vi "Set Path.vi"(7 "Use base-path?":bool, 8 "error in (no error)":errorcluster, 9 "Encode?":bool, 10 "path":string, 11 "URI in":refnum<class "URI.lvclass">) -> (0 "error out":errorcluster, 3 "URI out":refnum<class "URI.lvclass">)   [LabVIEW 2013, in "openURI.lvlib" / "URI.lvclass"]
uses:
  URI.lvclass
  URI.lvclass/URI.ctl
  utilities/isHEXDigit.vi
  components/path/Get base-path.vi
  components/path/Create Path (string).vi
  <vilib>/Utility/error.llb/Error Cluster From Error Code.vi
  checkCached.vi
  components/path/URI-Component.Path.lvclass
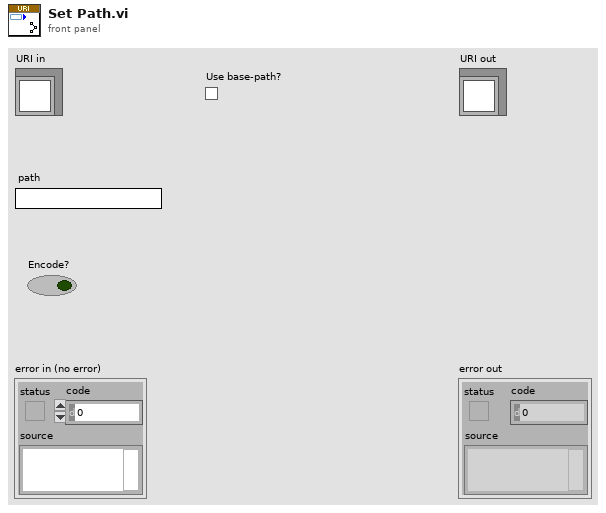
[diagram p1: front panel]
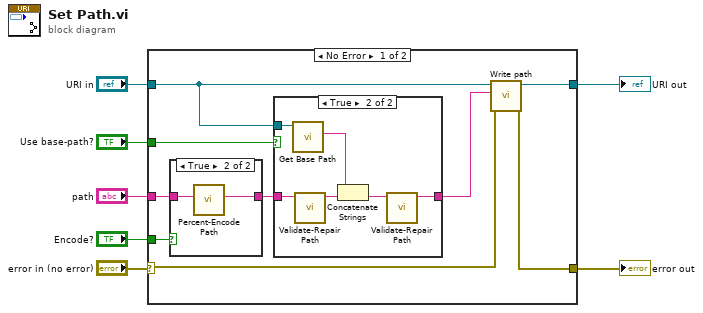
[diagram p0: block diagram]
diagram:
  n1 = case shown="No Error" "error in (no error)" {
    selector: "error in (no error)" -> [w13 w28]
    tunnel: [w12 w28] -> w6
    tunnel: [w16 w27] -> w4
    tunnel: "URI in" -> [w10 w27]
    tunnel: "path" -> [w14 _]
    tunnel: "Encode?" -> [w15 _]
    tunnel: "Use base-path?" -> [w11 _]
    frame No Error {
      n2 = case shown="True" w15 {
        tunnel: [w24 w25] -> w9
        tunnel: w14 -> [w24 w26]
        frame False {
        }
        frame True {
          n3 = call "Percent-Encode Path.vi"("Path"=w26) -> ("Pct-Encoded Path"=w25:string)  [unwired: 10 in]
        }
      }
      n4 = case shown="True" w11 {
        tunnel: w10 -> [_ w23]
        tunnel: w9 -> [w17 w22]
        tunnel: [w17 w21] -> w8
        frame False {
        }
        frame True {
          n5 = call "Get Base Path.vi"("URI in"=w23) -> ("base-path"=w19:string)  [unwired: 8 in, 2 out]
          n6 = call "Validate-Repair Path.vi"("path in"=w22) -> ("path out"=w18:string)  [unwired: 7 in, 3 out]
          n7 = Concatenate Strings(w19, w18) -> (w20:string)
          n8 = call "Validate-Repair Path.vi"("path in"=w20) -> ("path out"=w21:string)  [unwired: 7 in, 3 out]
        }
      }
      n9 = call "Write path.vi"("error in (no error)"=w13, "path"=w8, "URI in"=w10) -> ("error out"=w12:errorcluster, "URI out"=w16:refnum<class "URI.lvclass">)  [unwired: 7 in]
    }
    frame Error {
    }
  }
  "error out" <- w6
  "URI out" <- w4
